vi "Image_Pixel_Values_GCFS.vi"(4 "?":T1={"Core"={"Current VI Reference"=refnum, "Close Panel on Exit?"=FALSE}, "Camera Cluster"={"Session"="", "Image"=refnum, "Position Image"=refnum, "PixelVal Image"=refnum, "Position Image Binary"=refnum, "Lable Image"=refnum, "Merged Image"=refnum, "Connection"=FALSE}, "Data In Cluster"={"Images"={"Position Image path"=path "", "Sample folder path"=path "", "Label Image path"=path ""}, "Sample Name"="", "Sample Rate"=0, "Gradient Buffer"=0, "Data Acquisition.Setup.TempGrad"=0.0, "Control.PID gains"={"proportional gain (Kc)"=0.0, "integral time (Ti, min)"=0.0, "derivative time (Td, min)"=0.0}, "Freezing value"=250.0, "Sample Rate 2"=20}, "Active"=FALSE, "Ready"=FALSE, "Exit"=FALSE, "Arduino"={"Connection"=FALSE, "Port"="", "State"=""}, "Program_Start"="", "Data Out Cluster"={"Particle Measurements"=[], "Number of droplets"=0, "PosImg_Timestamp"="", "OverlayProp"=[], "Group"="", "Que"=refnum}, "PSU"={"Connection"=FALSE, "Port"="", "State"=""}, "Load Rerun"=FALSE, "Rerun"=FALSE, "cDAQ"={"Connection"=FALSE, "ID"="", "Task"=""}, "Temp"={"Manual Temp"=FALSE, "Target"=0.0}, "Cool A."=FALSE} {"Data Out Cluster"."Particle Measurements" format="%.2f"; "Data In Cluster"."Sample Rate 2" min=20 max=240 format="%.0f samples/min"}, 6 "date/time string":string, 7 "Image in":T3, 8 "Temperature":dbl format="%#_13g") -> (0 "error out":errorcluster, 1 "Value_Array":string[](array[string]), 2 "Freezing_points":string[](array[string]), 3 "Freezing data":bool)   [LabVIEW 2024]
uses:
  <vilib>/vision/Image Controls.llb/IMAQ Image.ctl
  Micro/DataCluster_GCFS.ctl
  <vilib>/userDefined/High Color/IMAQdx.ctl
  <vilib>/vision/Image Controls.llb/Overlay Property.ctl
  <vilib>/regexp/Match Regular Expression.xnode
  <vilib>/vision/NI_Vision_Development_Module.lvlib
panel:
  # "2,6 On INC_Old"
  # "0,08 On INC_Old"
  # "0,1 On INC_Old"
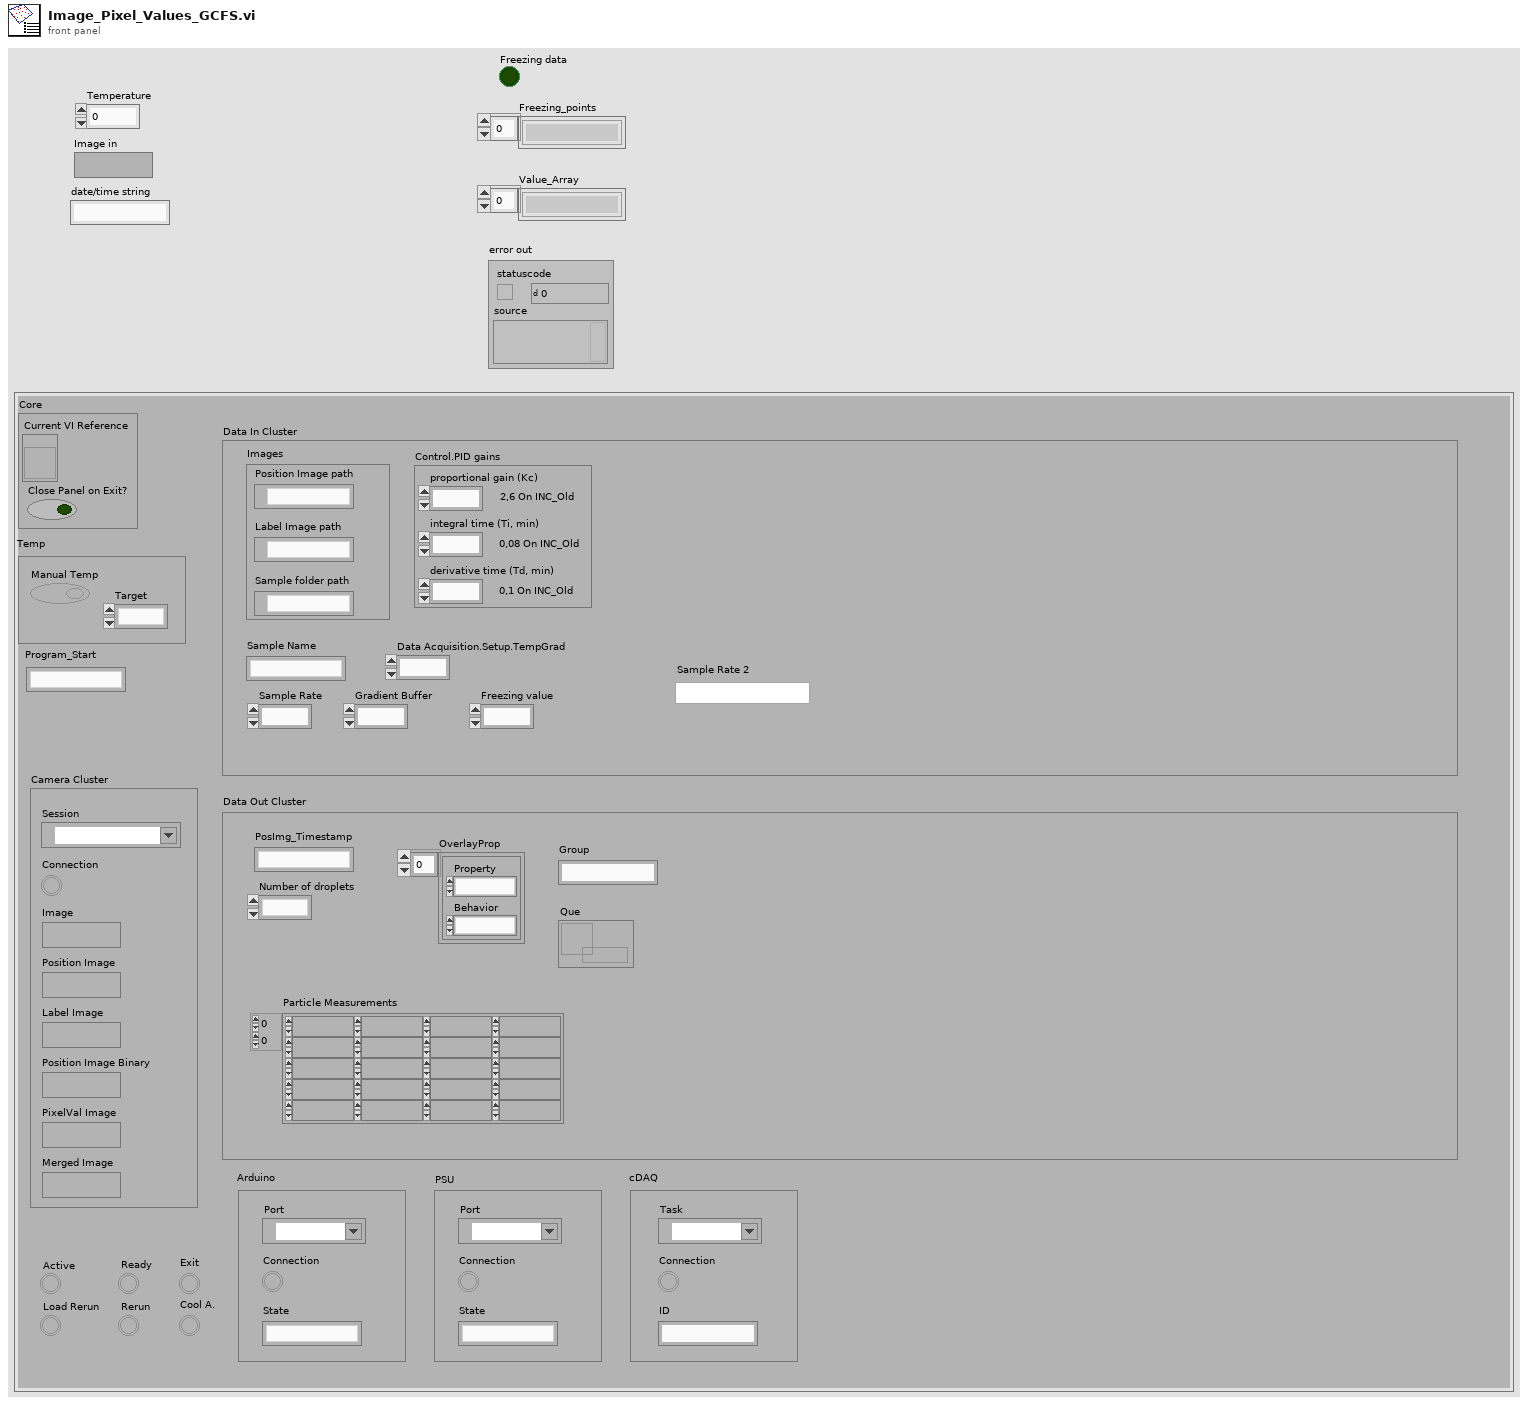
[diagram p1: front panel]
types:
  T1 = typedef "DataCluster_GCFS.ctl" = cluster{"Core":cluster{"Current VI Reference":refnum<vi>, "Close Panel on Exit?":bool}, "Camera Cluster":cluster{"Session":T2, "Image":T3, "Position Image":T3, "PixelVal Image":T3, "Position Image Binary":T3, "Lable Image":T3, "Merged Image":T3, "Connection":bool}, "Data In Cluster":cluster{"Images":cluster{"Position Image path":path, "Sample folder path":path, "Label Image path":path}, "Sample Name":string, "Sample Rate":i32, "Gradient Buffer":i32, "Data Acquisition.Setup.TempGrad":dbl, "Control.PID gains":cluster{"proportional gain (Kc)":dbl, "integral time (Ti, min)":dbl, "derivative time (Td, min)":dbl}, "Freezing value":sgl, "Sample Rate 2":i32}, "Active":bool, "Ready":bool, "Exit":bool, "Arduino":cluster{"Connection":bool, "Port":refnum<visa-resource-name>, "State":string}, "Program_Start":string, "Data Out Cluster":cluster{"Particle Measurements":dbl[][], "Number of droplets":i32, "PosImg_Timestamp":string, "OverlayProp":T4[], "Group":string, "Que":refnum<queue>}, "PSU":cluster{"Connection":bool, "Port":refnum<visa-resource-name>, "State":string}, "Load Rerun":bool, "Rerun":bool, "cDAQ":cluster{"Connection":bool, "ID":string, "Task":refnum<k21>}, "Temp":cluster{"Manual Temp":bool, "Target":dbl}, "Cool A.":bool}
  T2 = typedef "IMAQdx.ctl" = refnum<k21>
  T3 = typedef "IMAQ Image.ctl" = refnum<image>
  T4 = typedef "Overlay Property.ctl" = cluster{"Property":enum32{"Scale", "Shift", "Rotate", "Symmetry"}, "Behavior":enum32{"Clear", "Keep", "Transform"}}
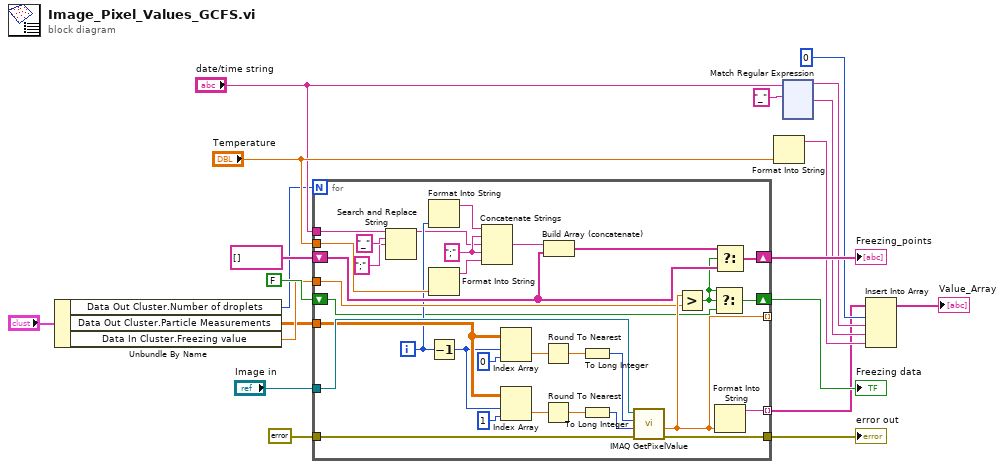
[diagram p0: block diagram]
diagram:
  n1 = Unbundle By Name("?") -> ("Data Out Cluster.Number of droplets"=w2:i32, "Data Out Cluster.Particle Measurements"=w3:dbl[][], "Data In Cluster.Freezing value"=w4:sgl)
  n2 = for {
    N: w2 -> [_]
    tunnel: "Image in" -> [w52]
    tunnel: [w48] -> _ mode=indexing
    tunnel: [w49] -> w10 mode=indexing
    tunnel: "date/time string" -> [w24]
    shift-right: [w47] -> w19
    shift-left: string[] [] -> [w43]
    tunnel: w4 -> [w42]
    tunnel: "Temperature" -> [w40]
    tunnel: w3 -> [w36]
    shift-right: [w28] -> w17
    shift-left: FALSE -> [w27]
    tunnel: errorcluster {"status"=FALSE, "code"=0, "source"=""} ("error in (no error)") -> [w26]
    tunnel: [w25] -> w6
    i -> [w35]
    w41 = ";" ("string")
    n3 = Search and Replace String(input string=w24, search string="_" ("input string"), replace string=";" ("replace string (\"\")")) -> (result string=w23:string)  [unwired: 5 in, 3 out]
    n4 = Format Into String(w35) -> (resulting string=w46:string)  [unwired: 3 in, 1 out]
    n5 = Format Into String(w40) -> (resulting string=w39:string)  [unwired: 3 in, 1 out]
    n6 = Decrement(x=w35) -> (x-1=w34:i32)
    n7 = Concatenate Strings(w46, w41, w23, w41, w39) -> (w45:string)
    n8 = Index Array(array=w36, index (row)=w34, index (col)=0 ("disabled index (col)")) -> (element=w30:dbl)
    n9 = Index Array(array=w36, index (row)=w34, index (col)=1) -> (element=w33:dbl)
    n10 = Round To Nearest(number=w30) -> (nearest integer value=w31:dbl)
    n11 = Round To Nearest(number=w33) -> (nearest integer value=w32:dbl)
    n12 = Build Array (concatenate)(w45, w43) -> (w44:string[])
    n13 = To Long Integer(number=w31) -> (32bit integer=w51:i32)
    n14 = To Long Integer(number=w32) -> (32bit integer=w50:i32)
    n15 = call "IMAQ GetPixelValue"("Image"=w52, "X Coordinate"=w51, "Y Coordinate"=w50, "error in (no error)"=w26) -> ("Pixel Value (Float)"=w48:sgl, "error out"=w25:errorcluster)  [unwired: 2 in, 3 out]
    n16 = Greater?(x=w48, y=w42) -> (0:w29:bool)
    n17 = Select(t=w29, s=w29, f=w27) -> (s? t:f=w28:bool)
    n18 = Select(t=w44, s=w29, f=w43) -> (s? t:f=w47:string[])
    n19 = Format Into String(w48) -> (resulting string=w49:string)  [unwired: 3 in, 1 out]
  }
  "Freezing_points" <- w19
  "Freezing data" <- w17
  "error out" <- w6
  n20 = Format Into String("Temperature") -> (resulting string=w11:string)  [unwired: 3 in, 1 out]
  n21 = xnode "Match Regular Expression"("input string"="date/time string", "regular expression"="_" ("search string/char (-)")) -> ("before match"=w12:string, "after match"=w13:string)  [unwired: 4 in, 3 out]
  n22 = Insert Into Array(array=w10, index=0, new element #1=w12, new element #2=w13, new element #3=w11) -> (→"Value_Array":string[])
